vi "NumericCtlCoercion.vi"() -> ()   [LabVIEW 2016]
panel:
  in  "Numeric":dbl=100.0 min=100.0 max=200.0
  in  "STOP":bool
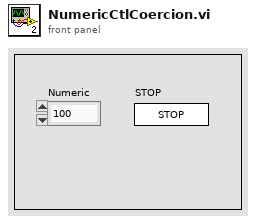
[diagram p1: front panel]
types:
  T1 = enum32{"Invalid", "Standard", "Closed", "Hidden", "Minimized", "Maximized"}
  T2 = enum32{"invalid app kind", "Development System", "Run Time System", "Student Edition", "Embedded LabVIEW", "Evaluation", "Custom"}
  T3 = cluster{"Core":cluster{"Current VI Reference":refnum<vi>, "Close Panel on Exit?":bool}, "Your Boolean data":bool, "Your string data":string}
  T4 = cluster{"Current VI Reference":refnum<vi>, "Close Panel on Exit?":bool}
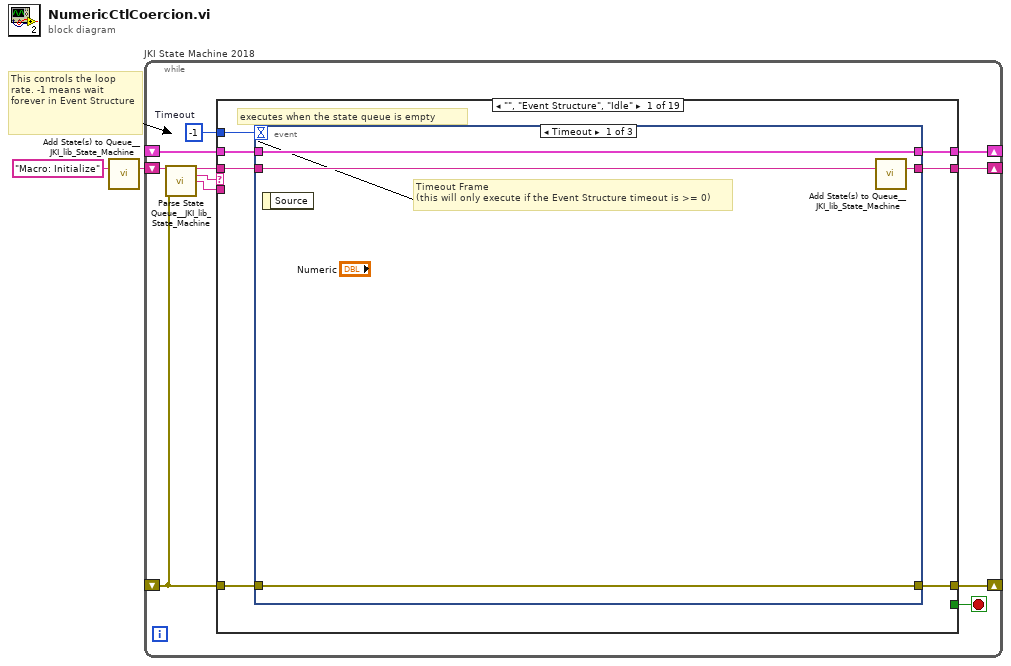
[diagram p0: block diagram]
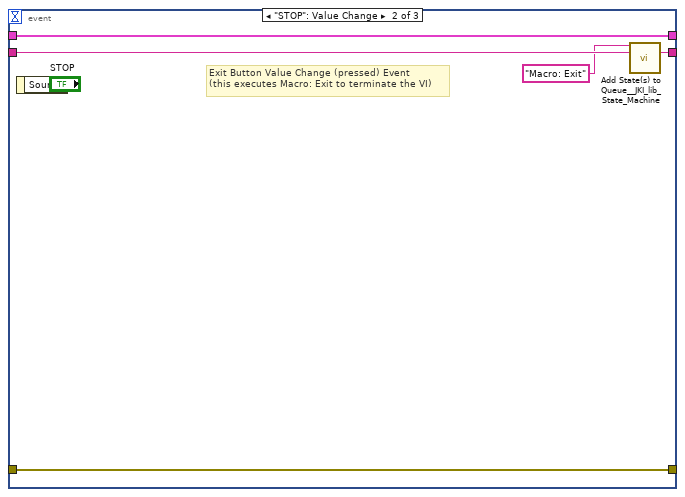
[diagram p2: hidden frame]
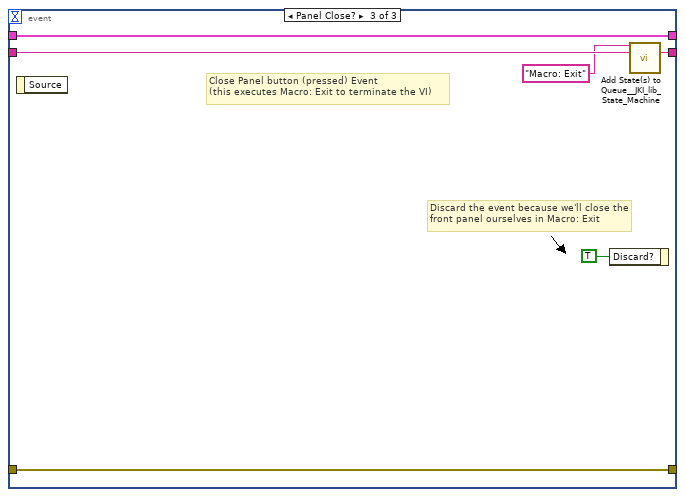
[diagram p3: hidden frame]
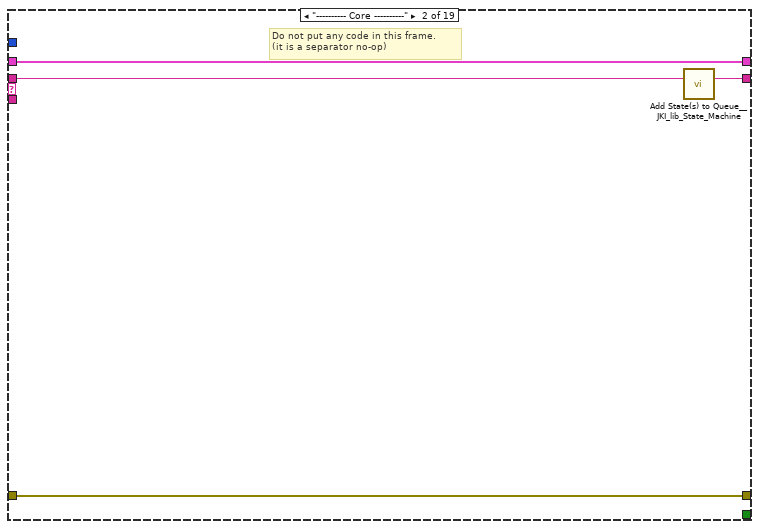
[diagram p4: hidden frame]
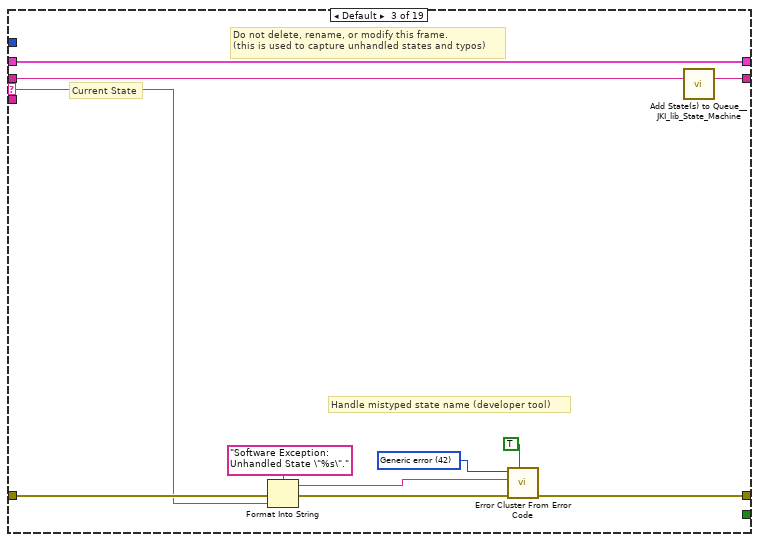
[diagram p5: hidden frame]
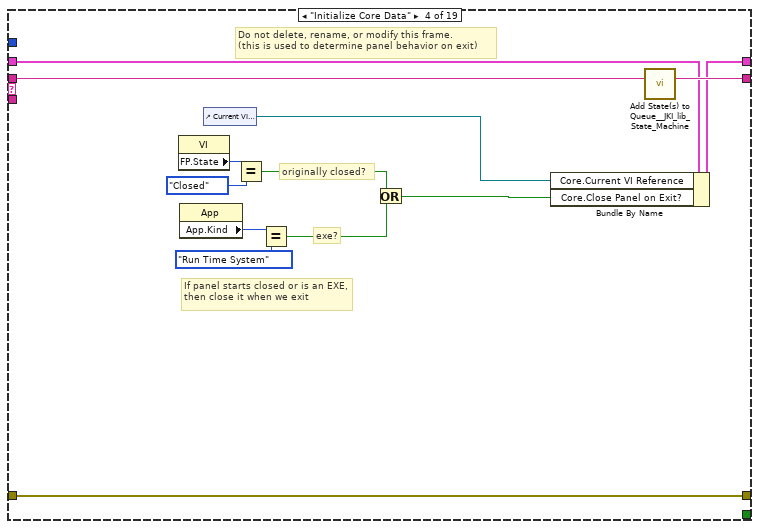
[diagram p6: hidden frame]
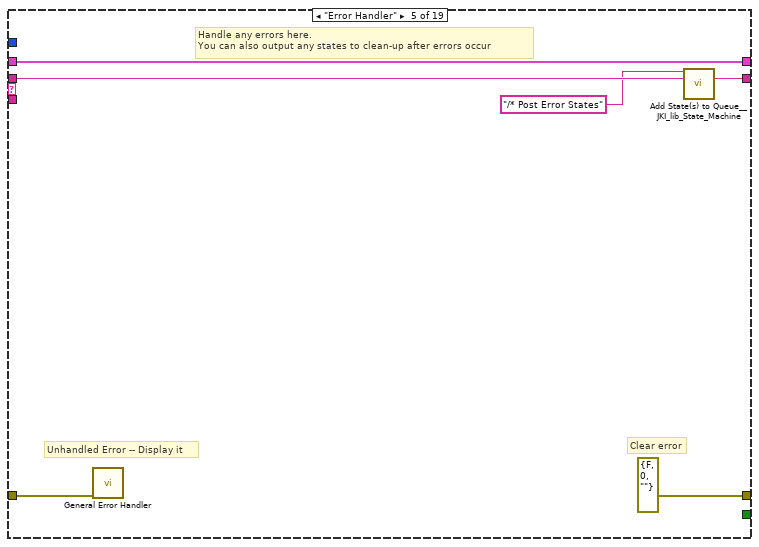
[diagram p7: hidden frame]
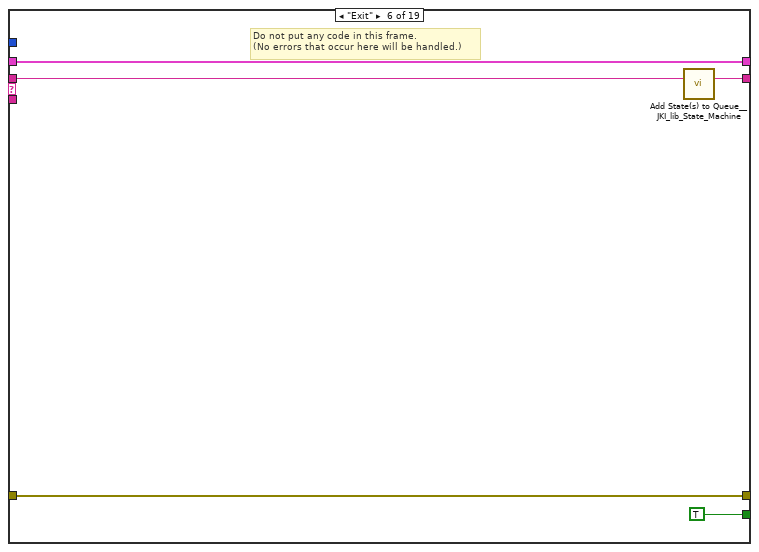
[diagram p8: hidden frame]
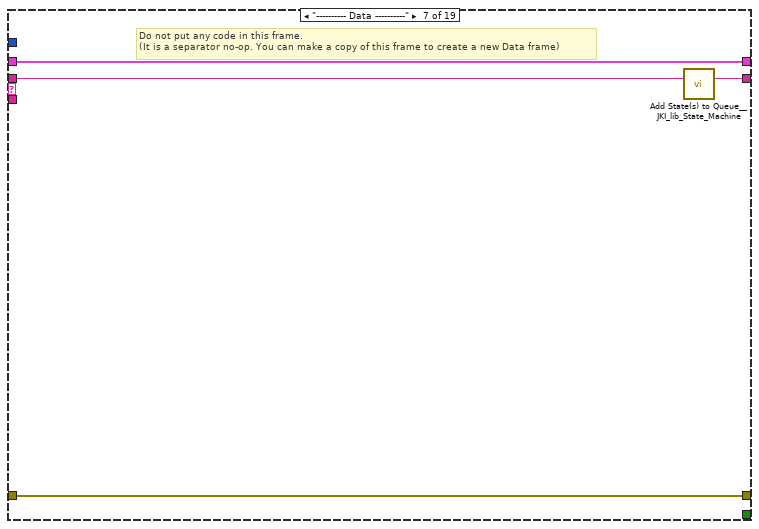
[diagram p9: hidden frame]
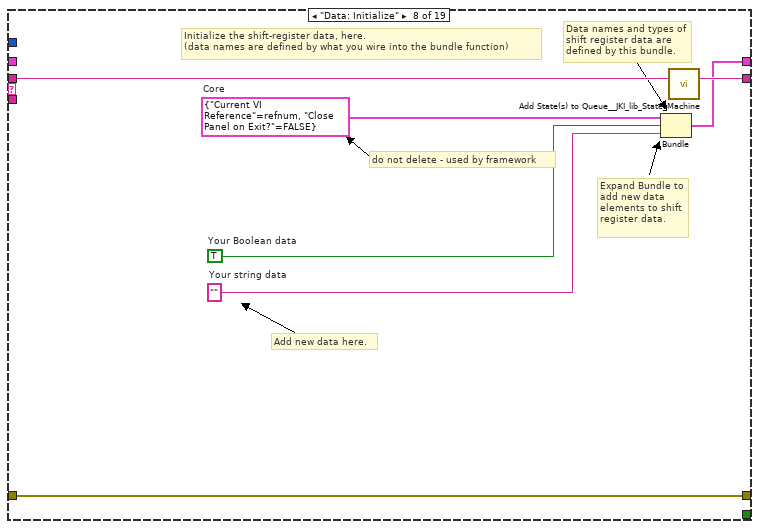
[diagram p10: hidden frame]
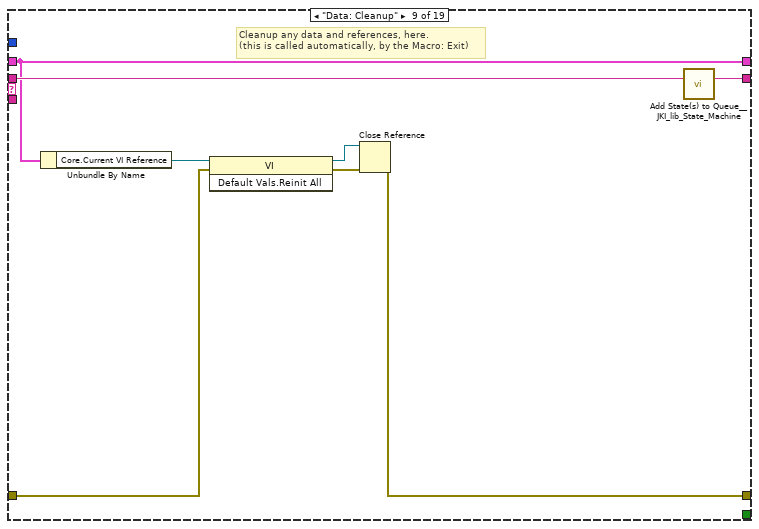
[diagram p11: hidden frame]
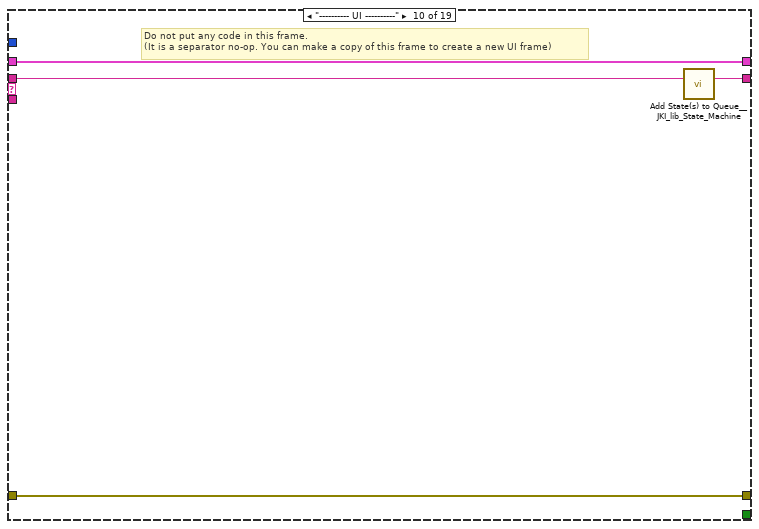
[diagram p12: hidden frame]
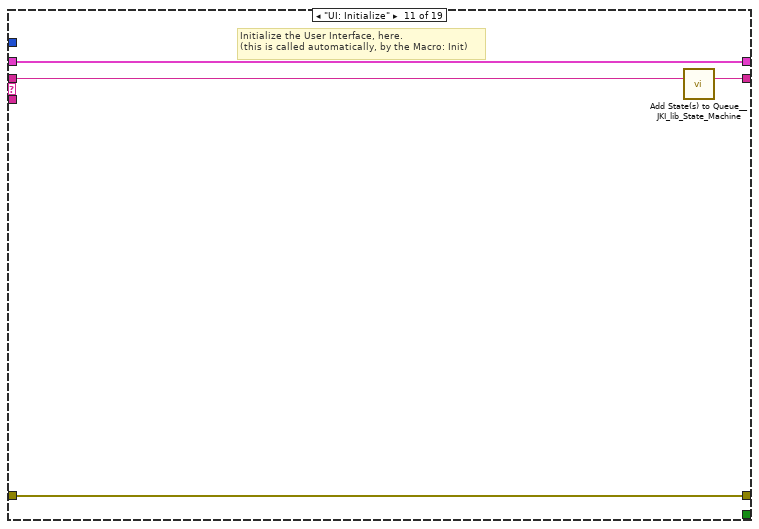
[diagram p13: hidden frame]
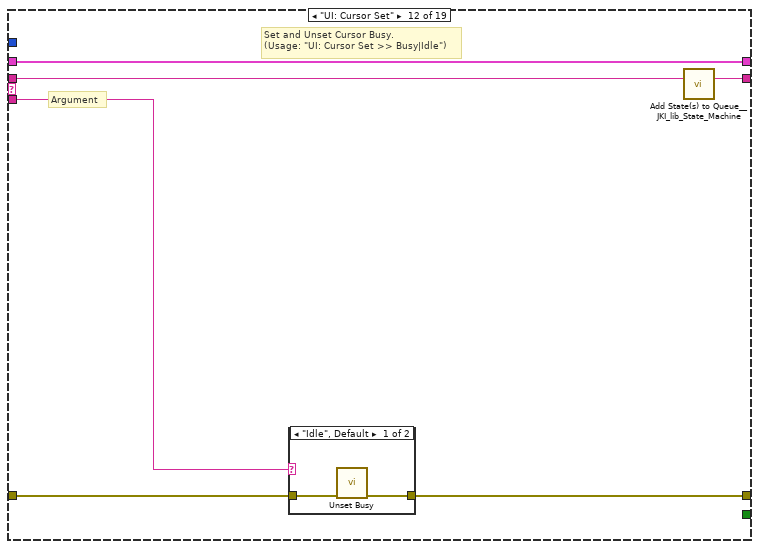
[diagram p14: hidden frame]
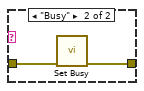
[diagram p15: hidden frame]
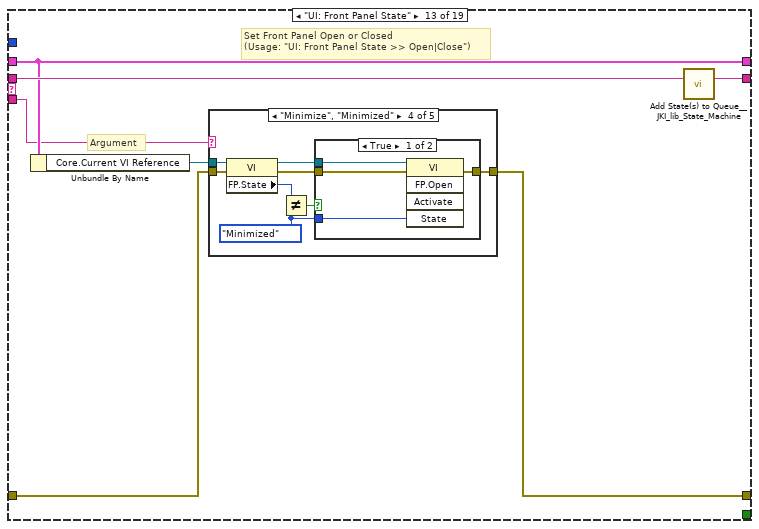
[diagram p16: hidden frame]
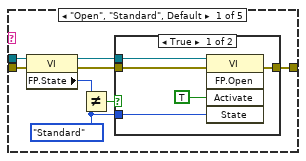
[diagram p17: hidden frame]
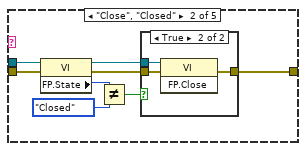
[diagram p19: hidden frame]
diagram:
  # "This controls the loop rate. -1 means wait forever in Event Structure"
  n1 = call <vilib>:"Add State(s) to Queue__JKI_lib_State_Machine.vi"("State(s) in (\"\")"="Macro: Initialize") -> ("States Out"=w2:string)  [unwired: 14 in]
  n2 = while "JKI State Machine 2018" {
    shift-right: [w6] -> _
    shift-left: _ -> [w5]
    shift-right: [w9] -> _
    shift-left: _ -> [w3]
    shift-right: [w8] -> _
    shift-left: w2 -> [w10]
    stop <- w7 stop-if-true
    w4 = -1  # Timeout
    n3 = call <vilib>:"Parse State Queue__JKI_lib_State_Machine.vi"("State Queue"=w10, "Error In (no error)"=w3) -> ("Remaining States"=w12:string, "Current State"=w13:string, "Arguments"=w11:string)  [unwired: 11 in]
    n4 = case shown="\"\", \"Event Structure\", \"Idle\"" w13 {
      selector: w13 -> [_ _ w40 _ _ _ _ _ _ _ _ _ _ _ _ _ _ _ _]
      tunnel: w12 -> [w20 w39 w44 w63 w69 w74 w78 w85 w93 w97 w101 w107 w118 w187 w192 w202 w206 w210 w214]
      tunnel: w11 -> [_ _ _ _ _ _ _ _ _ _ _ w102 w112 _ _ _ _ _ _]
      tunnel: w5 -> [w18 w36 w42 w56 w66 w72 w75 _ w90 w94 w99 w105 w114 w184 w189 w199 w203 w207 w211]
      tunnel: [w17 w37 w46 w60 errorcluster {"status"=FALSE, "code"=0, "source"=""} ("error out") w71 w76 w82 w91 w95 w98 w103 w115 w185 w190 w200 w204 w208 w212] -> w9
      tunnel: w3 -> [w16 w37 w45 w60 w65 w71 w76 w82 w86 w95 w98 w104 w116 w185 w190 w200 w204 w208 w212]
      tunnel: [w19 w38 w43 w62 w68 w73 w77 w84 w92 w96 w100 w106 w117 w186 w191 w201 w205 w209 w213] -> w8
      tunnel: [_ _ _ _ _ TRUE _ _ _ _ _ _ _ _ _ _ _ _ _] -> w7
      tunnel: [w15 w36 w42 w61 w66 w72 w75 w83 w90 w94 w99 w105 w114 w184 w189 w199 w203 w207 w211] -> w6
      tunnel: w4 -> [w14 _ _ _ _ _ _ _ _ _ _ _ _ _ _ _ _ _ _]
      frame "", "Event Structure", "Idle" {
        # "executes when the state queue is empty"
        n5 = event shown="[0] Timeout" {
          selector: _ -> [_ _ _]
          dyn-events: _ -> [_ _ _]
          timeout: w14 -> [_ _ _]
          tunnel: w20 -> [w24 w29 w35]
          tunnel: [w23 w28 w34] -> w19
          tunnel: w18 -> [w21 w26 w32]
          tunnel: [w22 w27 w33] -> w17
          tunnel: w16 -> [w22 w27 w33]
          tunnel: [w21 w26 w32] -> w15
          event Timeout {
            # "Timeout Frame\n(this will only execute if the Event Structure timeout is >= 0)"
            n6 = event-data() -> ()  [unwired: 1 in, 1 out]
            n7 = call <vilib>:"Add State(s) to Queue__JKI_lib_State_Machine.vi"("State(s) in (\"\")"=w24) -> ("States Out"=w23:string)  [unwired: 14 in]
          }
          event "STOP": Value Change {
            # "Exit Button Value Change (pressed) Event\n(this executes Macro: Exit to terminate the VI)"
            n8 = event-data() -> ()  [unwired: 1 in, 1 out]
            n9 = call <vilib>:"Add State(s) to Queue__JKI_lib_State_Machine.vi"("State(s) in Front (\"\")"="Macro: Exit", "State(s) in (\"\")"=w29) -> ("States Out"=w28:string)  [unwired: 13 in]
          }
          event Panel Close? {
            # "Discard the event because we'll close the front panel ourselves in Macro: Exit"
            # "Close Panel button (pressed) Event\n(this executes Macro: Exit to terminate the VI)"
            n10 = event-data() -> ()  [unwired: 1 in, 1 out]
            n11 = event-data("Discard?"=TRUE) -> ()  [unwired: 1 in, 1 out]
            n12 = call <vilib>:"Add State(s) to Queue__JKI_lib_State_Machine.vi"("State(s) in Front (\"\")"="Macro: Exit", "State(s) in (\"\")"=w35) -> ("States Out"=w34:string)  [unwired: 13 in]
          }
        }
      }
      frame "---------- Core ----------" {
        # "Do not put any code in this frame.\n(it is a separator no-op)"
        n13 = call <vilib>:"Add State(s) to Queue__JKI_lib_State_Machine.vi"("State(s) in (\"\")"=w39) -> ("States Out"=w38:string)  [unwired: 14 in]
      }
      frame Default {
        w49 = 42 items=["No error", "Argument error", "Memory is full", "Out of zone", "End of file", "File already open", "Generic file I/O error", "File not found", "File permission error", "Disk is full", "Duplicate path", "Too many files open", "System feature not enabled", "Resource file not found", "Cannot add resource", "Resource not found", "Image not found", "Image memory error", "Pen does not exist", "Config type invalid", "Config token not found", "Config parse error", "Config memory error", "Bad external code format", "Bad external code offset", "External code not present", "Null window", "Destroy window error", "Null menu", "Print aborted", "Bad print record", "Print driver error", "Windows error during printing", "Memory error during printing", "Print dialog error", "Generic print error", "Invalid device refnum", "Device not found", "Device parameter error", "Device unit error", "Cannot open device", "Device call aborted", "Generic error", "Cancelled by user", "Object ID too low", "Object ID too high", "Object not in heap", "Unknown heap", "Unknown object (invalid DefProc)", "Unknown object (DefProc not in table)", "Message out of range", "Invalid (null) method", "Unknown message", "Manager call not supported", "Bad address", "Network operation in progress", "Network operation timed out", "Connection is busy", "Network attribute not supported", "Network error", "Address in use", "System out of memory", "Connection aborted", "Connection refused", "Not connected", "Already connected", "Connection closed", "Initialization error (interapplication manager)", "Bad occurrence", "Wait on unbound occurrence handler", "Occurrence queue overflow", "Datalog type conflict", "Unused", "Unrecognized type (interapplication manager)", "Memory corrupt", "Failed to make temporary DLL", "Old CIN version", "Drag socket not found", "Failed to load drop-object", "Failed to register OLE object", "Failed to release OLE object", "Format specifier type mismatch", "Unknown format specifier", "Too few format specifiers", "Too many format specifiers", "Scan failed", "Newer CIN version", "Error converting to variant", "Runtime menu error", "Password tampered", "Variant attribute not found", "Incompatible variant data type", "Event data is not available", "Event Store is not present", "Occurrence is not found", "Event Queue is not created", "Event info is not available", "Refnum passed is NULL", "Error retrieving Class GUID", "Error retrieving CoClass GUID", "Error retrieving TypeLib GUID.", "Bad built application magic bytes.", "Specific driver is different from the specific driver associated with the Logical Name.", "There is no session opened to the class driver.", "Max Error", "MAX - Error with config objects", "MAX - Error loading configuration", "MAX - Group not supported"]
        # "Current State"
        # "Do not delete, rename, or modify this frame.\n(this is used to capture unhandled states and typos)"
        # "Handle mistyped state name (developer tool)"
        n14 = Format Into String(format string="Software Exception: Unhandled State \"%s\"." ("message"), error in=w45, w40) -> (resulting string=w48:string, error out=w47:errorcluster)  [unwired: 1 in]
        n15 = call <vilib>:"Error Cluster From Error Code.vi"("show call chain? (False)"=TRUE, "error in (no error)"=w47, "error message (\"\")"=w48, "error code (0)"=w49) -> ("error out"=w46:errorcluster)  [unwired: 5 in]
        n16 = call <vilib>:"Add State(s) to Queue__JKI_lib_State_Machine.vi"("State(s) in (\"\")"=w44) -> ("States Out"=w43:string)  [unwired: 14 in]
      }
      frame "Initialize Core Data" {
        # "Do not delete, rename, or modify this frame.\n(this is used to determine panel behavior on exit)"
        # "originally closed?"
        # "exe?"
        # "If panel starts closed or is an EXE, then close it when we exit"
        n17 = property class="VI"() -> ("FP.State"=w53:T1)  [unwired: 2 in, 2 out]
        n18 = property class="App"() -> ("App.Kind"=w59:T2)  [unwired: 2 in, 2 out]
        n19 = control-ref of="Current VI Reference"() -> (w54:refnum<vi>)
        n20 = Equal?(x=w53, y=T1."Closed" ("Front Panel Window:State")) -> (x = y?=w51:bool)
        n21 = Equal?(x=w59, y=T2."Run Time System" ("Application:Kind")) -> (x = y?=w57:bool)
        n22 = Or(x=w51, y=w57) -> (x .or. y?=w55:bool)
        n23 = Bundle By Name(cluster=w56, "Core.Current VI Reference"=w54, "Core.Close Panel on Exit?"=w55) -> (w61:T3)
        n24 = call <vilib>:"Add State(s) to Queue__JKI_lib_State_Machine.vi"("State(s) in (\"\")"=w63) -> ("States Out"=w62:string)  [unwired: 14 in]
      }
      frame "Error Handler" {
        # "Unhandled Error -- Display it"
        # "Handle any errors here.\nYou can also output any states to clean-up after errors occur"
        # "Clear error"
        n25 = call <vilib>:"General Error Handler.vi"("error in (no error)"=w65) -> ()  [unwired: 10 in, 5 out]
        n26 = call <vilib>:"Add State(s) to Queue__JKI_lib_State_Machine.vi"("State(s) in Front (\"\")"="/* Post Error States", "State(s) in (\"\")"=w69) -> ("States Out"=w68:string)  [unwired: 13 in]
      }
      frame "Exit" {
        # "Do not put any code in this frame.\n(No errors that occur here will be handled.)"
        n27 = call <vilib>:"Add State(s) to Queue__JKI_lib_State_Machine.vi"("State(s) in (\"\")"=w74) -> ("States Out"=w73:string)  [unwired: 14 in]
      }
      frame "---------- Data ----------" {
        # "Do not put any code in this frame.\n(It is a separator no-op. You can make a copy of this frame to create a new Data frame)"
        n28 = call <vilib>:"Add State(s) to Queue__JKI_lib_State_Machine.vi"("State(s) in (\"\")"=w78) -> ("States Out"=w77:string)  [unwired: 14 in]
      }
      frame "Data: Initialize" {
        w79 = T4 {"Current VI Reference"=refnum, "Close Panel on Exit?"=FALSE}  # Core
        w81 = TRUE  # Your Boolean data
        w80 = ""  # Your string data
        # "do not delete - used by framework"
        # "Expand Bundle to add new data elements to shift register data."
        # "Add new data here."
        # "Data names and types of shift register data are defined by this bundle."
        # "Initialize the shift-register data, here.\n(data names are defined by what you wire into the bundle function)"
        n29 = Bundle("Core"=w79, "Your Boolean data"=w81, "Your string data"=w80) -> (w83:T3)  [unwired: 1 in]
        n30 = call <vilib>:"Add State(s) to Queue__JKI_lib_State_Machine.vi"("State(s) in (\"\")"=w85) -> ("States Out"=w84:string)  [unwired: 14 in]
      }
      frame "Data: Cleanup" {
        # "Cleanup any data and references, here.\n(this is called automatically, by the Macro: Exit)"
        n31 = Unbundle By Name(w90) -> ("Core.Current VI Reference"=w89:refnum<vi>)
        n32 = invoke class="VI" method="Default Vals.Reinit All"(reference=w89, error in=w86) -> (reference out=w88:refnum<vi>, error out=w87:errorcluster)  [unwired: 1 in, 1 out]
        n33 = Close Reference(reference=w88, error in (no error)=w87) -> (error out=w91:errorcluster)
        n34 = call <vilib>:"Add State(s) to Queue__JKI_lib_State_Machine.vi"("State(s) in (\"\")"=w93) -> ("States Out"=w92:string)  [unwired: 14 in]
      }
      frame "---------- UI ----------" {
        # "Do not put any code in this frame.\n(It is a separator no-op. You can make a copy of this frame to create a new UI frame)"
        n35 = call <vilib>:"Add State(s) to Queue__JKI_lib_State_Machine.vi"("State(s) in (\"\")"=w97) -> ("States Out"=w96:string)  [unwired: 14 in]
      }
      frame "UI: Initialize" {
        # "Initialize the User Interface, here.\n(this is called automatically, by the Macro: Init)"
        n36 = call <vilib>:"Add State(s) to Queue__JKI_lib_State_Machine.vi"("State(s) in (\"\")"=w101) -> ("States Out"=w100:string)  [unwired: 14 in]
      }
      frame "UI: Cursor Set" {
        # "Argument"
        # "Set and Unset Cursor Busy.\n(Usage: \"UI: Cursor Set >> Busy|Idle\")"
        n37 = case shown="\"Idle\", Default" w102 {
          tunnel: w104 -> [w109 w111]
          tunnel: [w108 w110] -> w103
          frame "Idle", Default {
            n38 = call <vilib>:"Unset Busy.vi"("error in (no error)"=w109) -> ("error out"=w108:errorcluster)  [unwired: 10 in]
          }
          frame "Busy" {
            n39 = call <vilib>:"Set Busy.vi"("error in (no error)"=w111) -> ("error out"=w110:errorcluster)  [unwired: 9 in, 1 out]
          }
        }
        n40 = call <vilib>:"Add State(s) to Queue__JKI_lib_State_Machine.vi"("State(s) in (\"\")"=w107) -> ("States Out"=w106:string)  [unwired: 14 in]
      }
      frame "UI: Front Panel State" {
        # "Argument"
        # "Set Front Panel Open or Closed\n(Usage: \"UI: Front Panel State >> Open|Close\")"
        n41 = Unbundle By Name(w114) -> ("Core.Current VI Reference"=w113:refnum<vi>)
        n42 = case shown="\"Minimize\", \"Minimized\"" w112 {
          tunnel: w116 -> [w124 w139 w150 w163 w176]
          tunnel: [w126 w140 w152 w165 w178] -> w115
          tunnel: w113 -> [w125 w137 w151 w164 w177]
          frame "Open", "Standard", Default {
            w119 = T1."Standard" ("State")
            n43 = property class="VI"(reference=w125, error in=w124) -> (reference out=w122:refnum<vi>, error out=w123:errorcluster, "FP.State"=w121:T1)
            n44 = Not Equal?(x=w121, y=w119) -> (x != y?=w120:bool)
            n45 = case shown="True" w120 {
              tunnel: [w130 w132] -> w126
              tunnel: w123 -> [w129 w132]
              tunnel: w122 -> [w128 _]
              tunnel: w119 -> [w127 _]
              frame True {
                n46 = invoke class="VI" method="FP.Open"(reference=w128, error in=w129, "Activate"=TRUE, "State"=w127) -> (error out=w130:errorcluster)  [unwired: 1 in, 4 out]
              }
              frame False {
              }
            }
          }
          frame "Close", "Closed" {
            n47 = property class="VI"(reference=w137, error in=w139) -> (reference out=w136:refnum<vi>, error out=w138:errorcluster, "FP.State"=w134:T1)
            n48 = Not Equal?(x=w134, y=T1."Closed" ("Front Panel Window:State")) -> (x != y?=w133:bool)
            n49 = case shown="True" w133 {
              tunnel: [w141 w144] -> w140
              tunnel: w138 -> [w141 w143]
              tunnel: w136 -> [_ w142]
              frame False {
              }
              frame True {
                n50 = invoke class="VI" method="FP.Close"(reference=w142, error in=w143) -> (error out=w144:errorcluster)  [unwired: 1 in, 2 out]
              }
            }
          }
          frame "Hidden", "Hide" {
            w145 = T1."Hidden" ("State")
            n51 = property class="VI"(reference=w151, error in=w150) -> (reference out=w148:refnum<vi>, error out=w149:errorcluster, "FP.State"=w147:T1)
            n52 = Not Equal?(x=w147, y=w145) -> (x != y?=w146:bool)
            n53 = case shown="True" w146 {
              tunnel: [w156 w157] -> w152
              tunnel: w149 -> [w155 w157]
              tunnel: w148 -> [w154 _]
              tunnel: w145 -> [w153 _]
              frame True {
                n54 = invoke class="VI" method="FP.Open"(reference=w154, error in=w155, "State"=w153) -> (error out=w156:errorcluster)  [unwired: 2 in, 4 out]
              }
              frame False {
              }
            }
          }
          frame "Minimize", "Minimized" {
            w158 = T1."Minimized" ("State")
            n55 = property class="VI"(reference=w164, error in=w163) -> (reference out=w161:refnum<vi>, error out=w162:errorcluster, "FP.State"=w160:T1)
            n56 = Not Equal?(x=w160, y=w158) -> (x != y?=w159:bool)
            n57 = case shown="True" w159 {
              tunnel: [w169 w170] -> w165
              tunnel: w162 -> [w168 w170]
              tunnel: w161 -> [w167 _]
              tunnel: w158 -> [w166 _]
              frame True {
                n58 = invoke class="VI" method="FP.Open"(reference=w167, error in=w168, "State"=w166) -> (error out=w169:errorcluster)  [unwired: 2 in, 4 out]
              }
              frame False {
              }
            }
          }
          frame "Maximize", "Maximized" {
            w171 = T1."Maximized" ("State")
            n59 = property class="VI"(reference=w177, error in=w176) -> (reference out=w174:refnum<vi>, error out=w175:errorcluster, "FP.State"=w173:T1)
            n60 = Not Equal?(x=w173, y=w171) -> (x != y?=w172:bool)
            n61 = case shown="True" w172 {
              tunnel: [w182 w183] -> w178
              tunnel: w175 -> [w181 w183]
              tunnel: w174 -> [w180 _]
              tunnel: w171 -> [w179 _]
              frame True {
                n62 = invoke class="VI" method="FP.Open"(reference=w180, error in=w181, "State"=w179) -> (error out=w182:errorcluster)  [unwired: 2 in, 4 out]
              }
              frame False {
              }
            }
          }
        }
        n63 = call <vilib>:"Add State(s) to Queue__JKI_lib_State_Machine.vi"("State(s) in (\"\")"=w118) -> ("States Out"=w117:string)  [unwired: 14 in]
      }
      frame "---------- Macro ----------" {
        # "Do not put any code in this frame.\n(It is a separator no-op. You can make a copy of this frame to create a new Macro frame)"
        n64 = call <vilib>:"Add State(s) to Queue__JKI_lib_State_Machine.vi"("State(s) in (\"\")"=w187) -> ("States Out"=w186:string)  [unwired: 14 in]
      }
      frame "Macro: Initialize" {
        w188 = "Data: Initialize\nInitialize Core Data\nUI: Initialize\nUI: Front Panel State >> Open"  # Data: Initialize Initialize Core Data UI: Initialize UI: Front Panel State >> Open
        # "Initialization Macro\n(This is called once, when the VI starts)"
        n65 = call <vilib>:"Add State(s) to Queue__JKI_lib_State_Machine.vi"("State(s) in Front (\"\")"=w188, "State(s) in (\"\")"=w192) -> ("States Out"=w191:string)  [unwired: 13 in]
      }
      frame "Macro: Exit" {
        # "Exit Macro\n(This is called once, when the VI exits)"
        n66 = Unbundle By Name(w199) -> ("Core.Close Panel on Exit?"=w198:bool)
        n67 = Select(t="UI: Front Panel State >> Close", s=w198, f="") -> (s? t:f=w195:string)
        n68 = call <vilib>:"Add State(s) to Queue__JKI_lib_State_Machine.vi"("State(s) in (\"\")"=w195, "State(s) at Back (\"\")"="Data: Cleanup\nExit") -> ("States Out"=w193:string)  [unwired: 13 in]
        n69 = call <vilib>:"Add State(s) to Queue__JKI_lib_State_Machine.vi"("State(s) in Front (\"\")"=w193, "State(s) in (\"\")"=w202) -> ("States Out"=w201:string)  [unwired: 13 in]
      }
      frame "---------- New Category ----------" {
        # "Template Separator\n(You can make a copy of, or modify, this frame)"
        n70 = call <vilib>:"Add State(s) to Queue__JKI_lib_State_Machine.vi"("State(s) in (\"\")"=w206) -> ("States Out"=w205:string)  [unwired: 14 in]
      }
      frame "New Category: 1" {
        # "Your code here.\n(You can make a copy of, or modify, this frame)"
        n71 = call <vilib>:"Add State(s) to Queue__JKI_lib_State_Machine.vi"("State(s) in (\"\")"=w210) -> ("States Out"=w209:string)  [unwired: 14 in]
      }
      frame "New Category: 2" {
        # "Your code here.\n(You can make a copy of, or modify, this frame)"
        n72 = call <vilib>:"Add State(s) to Queue__JKI_lib_State_Machine.vi"("State(s) in (\"\")"=w214) -> ("States Out"=w213:string)  [unwired: 14 in]
      }
    }
  }
